vi "gfitsio-sizeof-cfitsio-datatype.vi"(11 "cfitsio datatype":T1 items=["TBIT"=1, "TBYTE  (U8)"=11, "TSBYTE  (I8)"=12, "TLOGICAL"=14, "TSTRING"=16, "TUSHORT  (U16)"=20, "TSHORT  (I16)"=21, "TUINT"=31, "TULONG  (U32)"=40, "TLONG  (I32)"=41, "TFLOAT  (SGL)"=42, "TLONGLONG  (I64)"=81, "TDOUBLE  (DBL)"=82, "TCOMPLEX  (CSG)"=83, "TDOUBLECOMPLEX  (CDB)"=163]) -> (1 "Variant datatype":variant, 2 "words/element":i32, 3 "size (bytes)":i32)   [LabVIEW 2014, in "gfitsio.lvlib"]
uses:
  gfitsio/gfitsio.lvlib
  cfitsio-datatypes.ctl
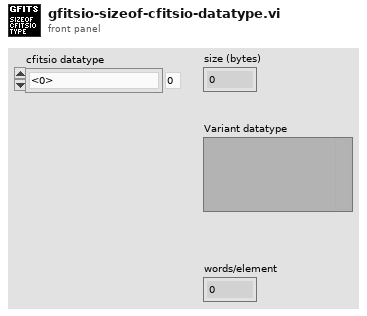
[diagram p1: front panel]
types:
  T1 = typedef "gfitsio.lvlib/cfitsio-datatypes.ctl" = i32
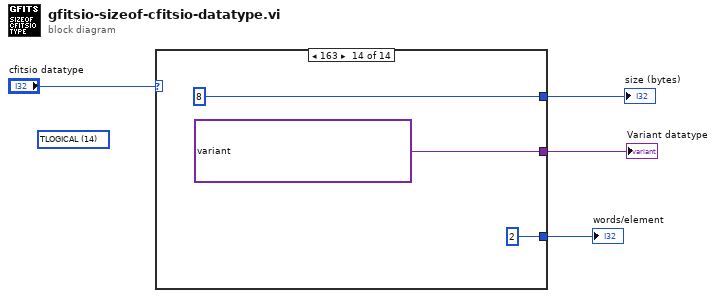
[diagram p0: block diagram]
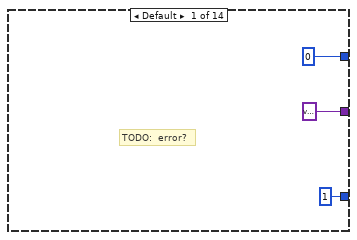
[diagram p2: hidden frame]
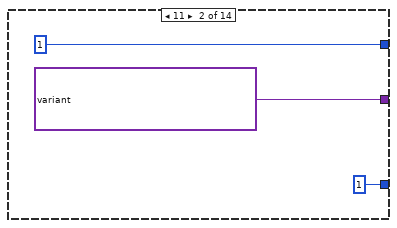
[diagram p3: hidden frame]
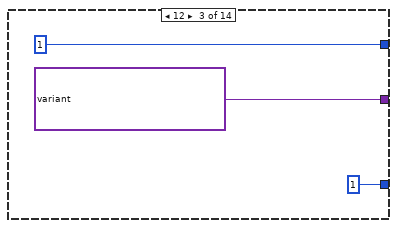
[diagram p4: hidden frame]
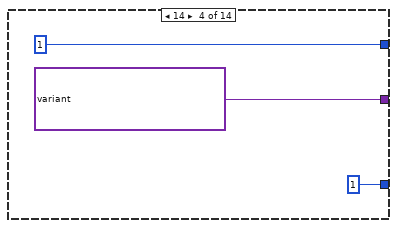
[diagram p5: hidden frame]
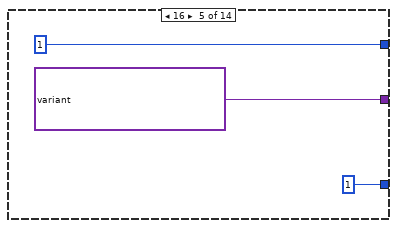
[diagram p6: hidden frame]
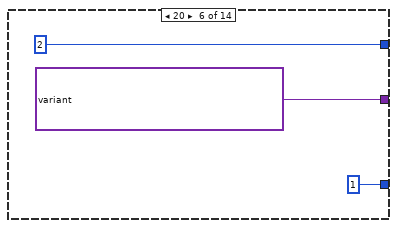
[diagram p7: hidden frame]
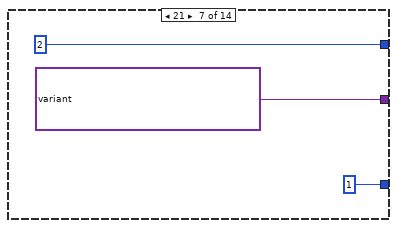
[diagram p8: hidden frame]
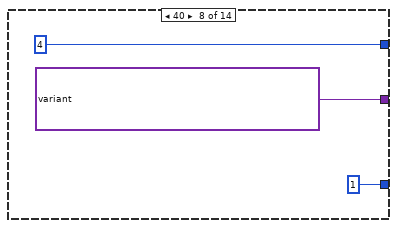
[diagram p9: hidden frame]
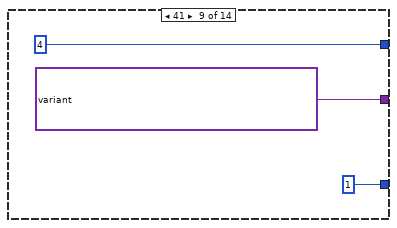
[diagram p10: hidden frame]
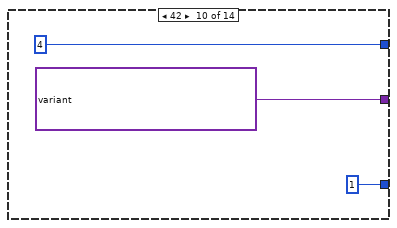
[diagram p11: hidden frame]
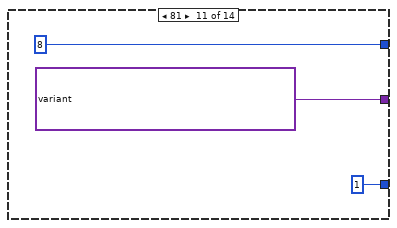
[diagram p12: hidden frame]
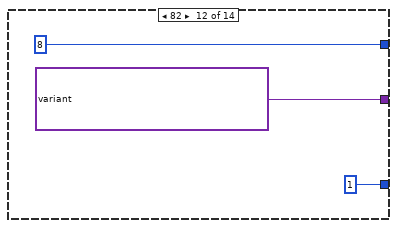
[diagram p13: hidden frame]
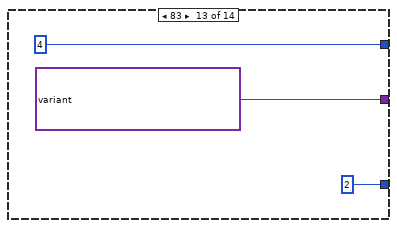
[diagram p14: hidden frame]
diagram:
  (unwired) T1 14 items=["TBIT"=1, "TBYTE  (U8)"=11, "TSBYTE  (I8)"=12, "TLOGICAL"=14, "TSTRING"=16, "TUSHORT  (U16)"=20, "TSHORT  (I16)"=21, "TUINT"=31, "TULONG  (U32)"=40, "TLONG  (I32)"=41, "TFLOAT  (SGL)"=42, "TLONGLONG  (I64)"=81, "TDOUBLE  (DBL)"=82, "TCOMPLEX  (CSG)"=83, "TDOUBLECOMPLEX  (CDB)"=163] ("cfitsio datatype")
  n1 = case shown="163" "cfitsio datatype" {
    tunnel: [0 1 1 1 1 2 2 4 4 4 8 8 4 8] -> w3
    tunnel: [variant ("variant") variant(u8 0) ("variant") variant(i8 0) ("variant") variant(bool FALSE) ("variant") variant(string "") ("variant") variant(u16 0) ("variant") variant(i16 0) ("variant") variant(u32 0) ("variant") variant(i32 0) ("variant") variant(sgl 0.0) ("variant") variant(i64 0) ("variant") variant(dbl 0.0) ("variant") variant(csg 0.0+0.0i) ("variant") variant(cdb 0.0+0.0i) ("variant")] -> w2
    tunnel: [1 ("words/element") 1 ("words/element") 1 ("words/element") 1 ("words/element") 1 ("words/element") 1 ("words/element") 1 ("words/element") 1 ("words/element") 1 ("words/element") 1 ("words/element") 1 ("words/element") 1 ("words/element") 2 ("words/element") 2 ("words/element")] -> w1
    frame Default {
      # "TODO:  error?"
    }
    frame 11 {
    }
    frame 12 {
    }
    frame 14 {
    }
    frame 16 {
    }
    frame 20 {
    }
    frame 21 {
    }
    frame 40 {
    }
    frame 41 {
    }
    frame 42 {
    }
    frame 81 {
    }
    frame 82 {
    }
    frame 83 {
    }
    frame 163 {
    }
  }
  "size (bytes)" <- w3
  "Variant datatype" <- w2
  "words/element" <- w1
